vi "Table, Set Active Cell.vi"(6 "error in":errorcluster, 7 "col (0)":i32, 8 "row (0)":i32, 9 "Tbl Refnum":refnum<vi>) -> (0 "error out":errorcluster, 3 "Tbl Refnum out":refnum<vi>)   [LabVIEW 2010]
doc: "Sets the active table cell."
uses:
  <vilib>/Utility/miscctls.llb/LVRowAndColumnTypeDef.ctl
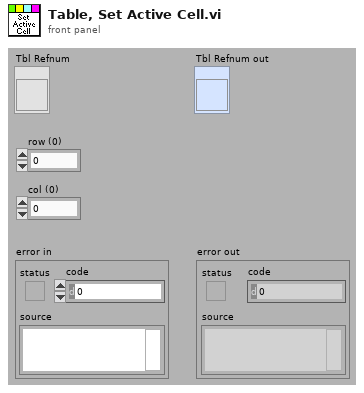
[diagram p1: front panel]
types:
  T1 = typedef "LVRowAndColumnTypeDef.ctl" = cluster{"Row":i32, "Column":i32}
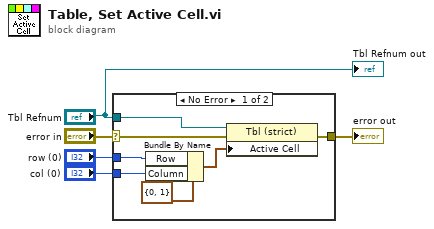
[diagram p0: block diagram]
diagram:
  n1 = case shown="No Error" "error in" {
    selector: "error in" -> [w9 w13]
    tunnel: [w12 w13] -> w5
    tunnel: "Tbl Refnum" -> [w11 _]
    tunnel: "row (0)" -> [w7 _]
    tunnel: "col (0)" -> [w6 _]
    frame No Error {
      n2 = Bundle By Name(cluster=T1 {"Row"=0, "Column"=1} ("Selection Start 2"), "Row"=w7, "Column"=w6) -> (w8:T1)
      n3 = property class="Tbl (strict)"(reference=w11, error in=w9, "Active Cell"=w8) -> (error out=w12:errorcluster)  [unwired: 1 out]
    }
    frame Error {
    }
  }
  "error out" <- w5
  "Tbl Refnum out" <- "Tbl Refnum"
